vi "AE Lunch.vi"(11 "Array of AEs":T1=[{"Name"="Peng", "Go?"=TRUE, "Which batch?"=enum."Anything"}, {"Name"="Xue Sheng", "Go?"=TRUE, "Which batch?"=enum."Anything"}, {"Name"="Denny", "Go?"=TRUE, "Which batch?"=enum."Anything"}, {"Name"="Wilbur", "Go?"=TRUE, "Which batch?"=enum."Anything"}, {"Name"="Hafiz", "Go?"=TRUE, "Which batch?"=enum."Anything"}, {"Name"="James", "Go?"=TRUE, "Which batch?"=enum."Anything"}, {"Name"="Sharath", "Go?"=TRUE, "Which batch?"=enum."Anything"}, {"Name"="Habib", "Go?"=TRUE, "Which batch?"=enum."Anything"}, {"Name"="Stephen", "Go?"=TRUE, "Which batch?"=enum."Anything"}]) -> (1 "Second Batch":string[](array[string])=["Peng", "Wilbur", "Hafiz", "James"], 2 "First Batch":string[](array[string])=["Xue Sheng", "Denny", "Habib"], 3 "String Return":string)   [LabVIEW 2016]
uses:
  Array AE Data.ctl
  AE Data.ctl
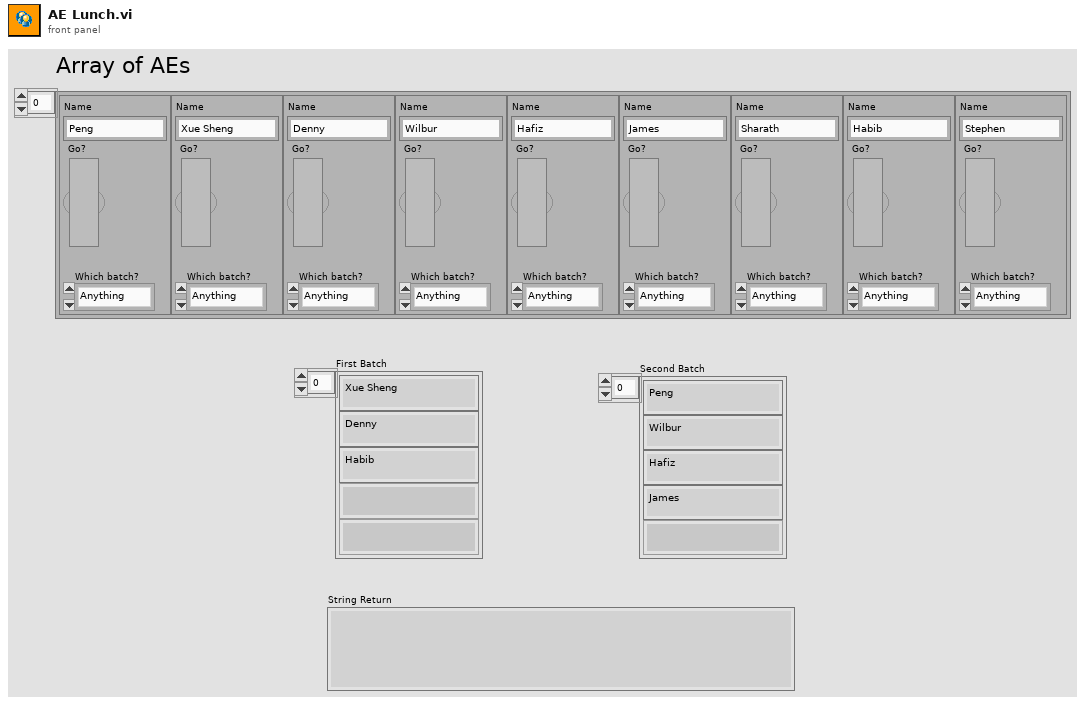
[diagram p1: front panel]
types:
  T1 = typedef "Array AE Data.ctl" = T2[]
  T2 = typedef "AE Data.ctl" = cluster{"Name":string, "Go?":bool, "Which batch?":enum16{"Anything", "First", "Second"}}
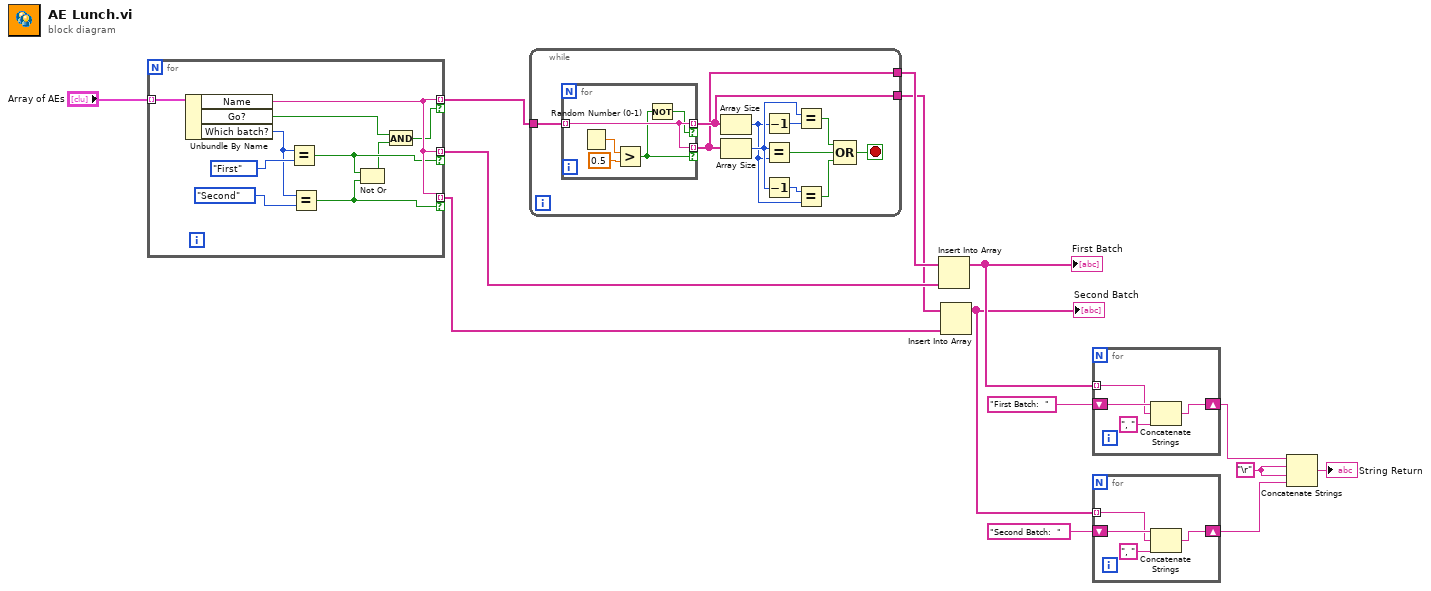
[diagram p0: block diagram]
diagram:
  w3 = "\r"
  n1 = for {
    tunnel: "Array of AEs" -> [w24] mode=indexing
    tunnel: [w20] -> w13 mode=indexing if=w15
    tunnel: [w20] -> w11 mode=indexing if=w19
    tunnel: [w20] -> w9 mode=indexing if=w18
    n2 = Unbundle By Name(w24) -> ("Name"=w20:string, "Go?"=w16:bool, "Which batch?"=w22:enum16{"Anything", "First", "Second"})
    n3 = Equal?(x=w22, y=enum16{"Anything", "First", "Second"}."First" ("Which batch?")) -> (x = y?=w19:bool)
    n4 = Equal?(x=w22, y=enum16{"Anything", "First", "Second"}."Second" ("Which batch?")) -> (x = y?=w18:bool)
    n5 = Not Or(1:w18, 2:w19) -> (0:w17:bool)
    n6 = And(x=w16, y=w17) -> (x .and. y?=w15:bool)
  }
  n7 = while {
    tunnel: [w35] -> w10
    tunnel: w13 -> [w34]
    tunnel: [w33] -> w12
    stop <- w31 stop-if-true
    n8 = for {
      tunnel: w34 -> [w38] mode=indexing
      tunnel: [w38] -> w33 mode=indexing if=w37
      tunnel: [w38] -> w35 mode=indexing if=w36
      n9 = Random Number (0-1)() -> (number: 0 to 1=w40:dbl)
      n10 = Greater?(x=w40, y=0.5) -> (0:w37:bool)
      n11 = Not(x=w37) -> (.not. x?=w36:bool)
    }
    n12 = Array Size(array=w35) -> (size(s)=w28:i32)
    n13 = Array Size(array=w33) -> (size(s)=w30:i32)
    n14 = Decrement(x=w28) -> (x-1=w32:i32)
    n15 = Equal?(x=w30, y=w28) -> (x = y?=w26:bool)
    n16 = Decrement(x=w30) -> (x-1=w29:i32)
    n17 = Equal?(x=w30, y=w32) -> (x = y?=w27:bool)
    n18 = Equal?(x=w29, y=w28) -> (x = y?=w25:bool)
    n19 = Compound Arithmetic op=OR(w27, w26, w25) -> (w31:bool)
  }
  n20 = Insert Into Array(array=w12, new element=w11) -> (w8:string[])  [unwired: 1 in]
  "First Batch" <- w8
  n21 = Insert Into Array(array=w10, new element=w9) -> (w5:string[])  [unwired: 1 in]
  "Second Batch" <- w5
  n22 = for {
    tunnel: w8 -> [w43] mode=indexing
    shift-right: [w41] -> w4
    shift-left: "First Batch:  " -> [w44]
    n23 = Concatenate Strings(w44, w43, ", ") -> (w41:string)
  }
  n24 = for {
    tunnel: w5 -> [w47] mode=indexing
    shift-right: [w45] -> w2
    shift-left: "Second Batch:  " -> [w48]
    n25 = Concatenate Strings(w48, w47, ", ") -> (w45:string)
  }
  n26 = Concatenate Strings(w4, w3, w3, w2) -> (→"String Return":string)
